vi "Event Number to Timestamp.vi"(1 "Event Number":i32) -> (0 "TimeStamp":string)   [LabVIEW 2010]
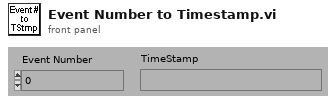
[diagram p1: front panel]
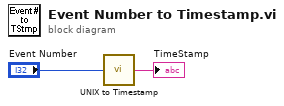
[diagram p0: block diagram]
diagram:
  n1 = call "UNIX to Timestamp.vi"("Seconds"="Event Number") -> ("Timestamp String"=→"TimeStamp":string)
